vi "Update Color Array.vi"(9 "Color Delta":T1={"Red"=0.0, "Green"=0.0, "Blue"=1.0, "Alpha"=1.0}, 10 "Current Index":i32, 11 "Color Array":cluster{dbl, dbl, dbl, dbl}[](array[cluster])) -> (3 "Updated Color":cluster{dbl, dbl, dbl, dbl}[](array[cluster]))   [LabVIEW 2014, in "Trajectory Drawer.lvclass"]
uses:
  Trajectory Drawer.lvclass
  <vilib>/Utility/miscctls.llb/LVRGBAColorTypeDef.ctl
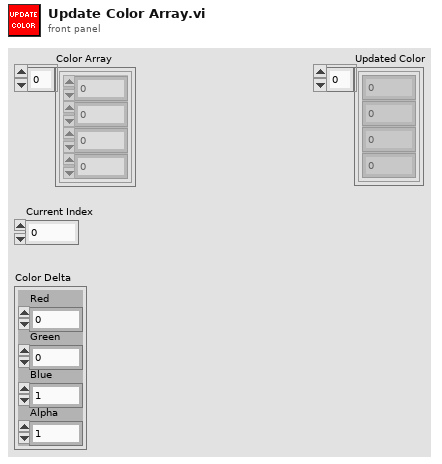
[diagram p1: front panel]
types:
  T1 = typedef "LVRGBAColorTypeDef.ctl" = cluster{"Red":sgl, "Green":sgl, "Blue":sgl, "Alpha":sgl}
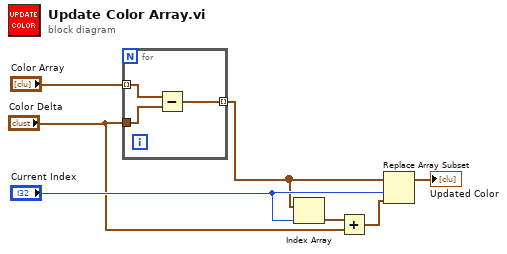
[diagram p0: block diagram]
diagram:
  n1 = for {
    tunnel: "Color Array" -> [w10] mode=indexing
    tunnel: "Color Delta" -> [w9]
    tunnel: [w8] -> w2 mode=indexing
    n2 = Subtract(x=w10, y=w9) -> (x-y=w8:cluster{dbl, dbl, dbl, dbl})
  }
  n3 = Index Array(array=w2, index="Current Index") -> (element=w1:cluster{dbl, dbl, dbl, dbl})
  n4 = Add(x=w1, y="Color Delta") -> (x+y=w7:cluster{dbl, dbl, dbl, dbl})
  n5 = Replace Array Subset(array=w2, new element=w7, index="Current Index") -> (→"Updated Color":cluster{dbl, dbl, dbl, dbl}[])
